vi "PH_Timing.Update Status.vi"(0 "i ref in":refnum<vi>, 5 "error in (no error)":errorcluster) -> (14 "i ref out":refnum<vi>, 19 "error out":errorcluster)   [LabVIEW 2014, in "PH_Timing.lvlib"]
doc: "By this VI the status of the timing instance is calculated, written to own attributes and published as DIM service. Additionally other services are updated.\n\n0 (no info): one or more child instances missed\n1 (off): instance started, all child instances available\n2 (on): ready to shot\n\nAdditionally the GUI elements are set."
uses:
  PH_Timing.lvlib
  PH_Basics/PH_StatusHandler/PH_StatusHandler.Status.ctl
  PH_Basics/PH_StatusHandler/PH_StatusHandler.lvlib
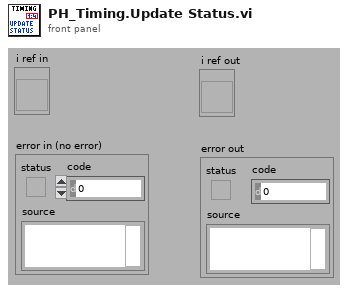
[diagram p1: front panel]
types:
  T1 = enum16{"Normal", "Single", "Burst", "Duty Cycle"}
  T2 = typedef "PH_StatusHandler.lvlib/PH_StatusHandler.Status.ctl" = i16
  T3 = typedef "PH_Timing.lvlib/PH_Timing.i attribute.ctl" = cluster{"Sequencer":cluster{"linked?":bool, "Proc State":string, "Ref State":refnum<vi>}, "Gate Generator":cluster{"GD":cluster{"Device Status":T2, "linked?":bool}, "Settings":T4, "GUI Ref":refnum<vi>}, "Interlock Bypass":cluster{"Instancename":string, "Switch linked?":bool, "Device Status":T2, "Ref Status":refnum<vi>}, "Roughtuner":cluster{"Settings":T5, "GUI Ref":refnum<vi>, "GD":cluster{"Device Status":T2, "linked?":bool}}, "0,5Hz Gater":cluster{"Settings":T6, "GUI Ref":refnum<vi>, "GD":cluster{"Device Status":T2, "linked?":bool}}, "Slow Trigger":cluster{"Settings":T7, "GUI Ref":refnum<vi>, "Service ID Delay":i32, "Service ID Ext Trig":i32, "Wanted Settings":T7}, "Timing Mode":cluster{"Mode":T8, "GUI Ref":refnum<vi>, "Service ID T2":i32, "Service ID Mode":i32, "Wanted Mode":T8}, "ns Generator":cluster{"Settings":T9, "ns Generator Settings":refnum<vi>, "GD":cluster{"Device Status":T2, "linked?":bool}}, "Phase FEs":cluster{"Settings":T12, "GUI Ref":refnum<vi>, "Service ID Phase":i32, "Wanted Settings":T12}, "GD GUI Refs":refnum<vi>[], "Heads":T13[], "GUI Ref Delete":refnum<vi>}
  T4 = typedef "PH_Timing.lvlib/PH_Timing.GateGen.ctl" = cluster{"Instance":string, "Channel Gate":i32, "Channel T2":i32, "Width Gate":dbl, "Width T2":dbl, "Delay Gate":dbl, "Delay T2":dbl, "Gate activ":bool, "T2 activ":bool, "System Mode":enum16{"Normal", "Single", "Burst", "Duty Cycle"}}
  T5 = typedef "PH_Timing.lvlib/PH_Timing.Roughtuner.ctl" = cluster{"Instance":string, "Phase PHELIX / UNILAC":cluster{"Channel":u16, "relative to":u16, "Delay [ms]":dbl}, "Pulse Length":cluster{"Channel":u16, "relative to":u16, "Delay [ms]":dbl}, "Trigger":cluster{"externally?":bool, "Rate [Hz]":dbl}}
  T6 = typedef "PH_Timing.lvlib/PH_Timing.0.5HzGater.ctl" = cluster{"Instance":string, "Channel ns FE Delay":i32, "Channel 0.5Hz":i32, "Width ns FE Delay":dbl, "Width 0.5Hz":dbl, "Delay ns FE Delay":dbl, "Delay 0.5Hz":dbl, "ns FE Delay active":bool, "0.5Hz activ":bool, "ns FE Delay inverted":bool, "0.5Hz inverted":bool}
  T7 = typedef "PH_Timing.lvlib/PH_Timing.Slow Trigger Settings.ctl" = cluster{"Delay":dbl, "externally triggered?":bool}
  T8 = typedef "PH_Timing.lvlib/PH_Timing.Timing Mode.ctl" = cluster{"T2":i16, "Modeselector":enum32{"10 Hz", "0.5 Hz", "Shot"}}
  T9 = typedef "PH_Timing.lvlib/PH_Timing.ns Generator.ctl" = cluster{"Instance":string, "Phase fs / ns FE":cluster{"Channel":T10, "Settings":T11}}
  T10 = typedef "Stanford Research DG645 - Driver.lvlib/Channel.ctl" = i32
  T11 = typedef "PH_SRDG645.lvlib/PH_SRDG645.Channel Settings.ctl" = cluster{"Delay [s]":dbl, "relative to":i32}
  T12 = typedef "PH_Timing.lvlib/PH_Timing.Phase FEs.ctl" = cluster{"Phase":dbl}
  T13 = typedef "PH_Timing.lvlib/PH_Timing.PU Data.ctl" = cluster{"linked?":bool, "Data":T14, "GD":cluster{"Device Status":T2, "linked?":bool}, "GUI Ref":refnum<vi>, "PU":T15}
  T14 = typedef "PH_Timing.lvlib/PH_Timing.PU Info.ctl" = cluster{"Act CH?":bool, "GD":string, "CH":i32, "Delay":dbl, "active":bool, "in Use?":bool}
  T15 = typedef "PH_PP_Common.lvlib/PH_PP_Common.PUs.ctl" = enum16{"no Info", "PA-19mm-1", "PA-19mm-2", "PA-45mm-PILC", "PA-45mm-MAIN", "MA-PU-1", "MA-PU-2", "MA-PU-3", "MA-PU-4", "MA-PU-5", "MA-PU-6", "MA-FR", "MA-PILC", "PA-45mm-DP"}
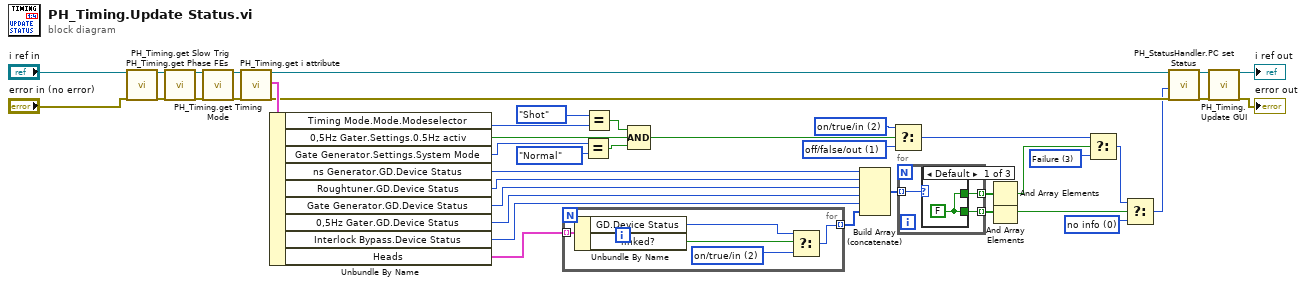
[diagram p0: block diagram]
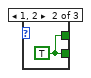
[diagram p2: hidden frame]
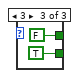
[diagram p3: hidden frame]
diagram:
  w21 = T2 1 items=["no info", "off/false/out", "on/true/in", "Failure", "Alarm", "Status 1", "Status 2", "Status 3"] ("Status.Device Status")
  w26 = T2 3 items=["no info", "off/false/out", "on/true/in", "Failure", "Alarm", "Status 1", "Status 2", "Status 3"] ("Status.Device Status")
  w23 = T2 2 items=["no info", "off/false/out", "on/true/in", "Failure", "Alarm", "Status 1", "Status 2", "Status 3"] ("Status.Device Status")
  w29 = T2 0 items=["no info", "off/false/out", "on/true/in", "Failure", "Alarm", "Status 1", "Status 2", "Status 3"] ("Status.Device Status")
  n1 = call "PH_Timing.get Phase FEs.vi"("i ref in"="i ref in", "error in"="error in (no error)") -> ("i ref out"=w32:refnum<vi>, "error out"=w31:errorcluster)  [unwired: 16 in]
  n2 = call "PH_Timing.get Slow Trig.vi"("i ref in"=w32, "error in"=w31) -> ("i ref out"=w36:refnum<vi>, "error out"=w34:errorcluster)  [unwired: 16 in]
  n3 = call "PH_Timing.get Timing Mode.vi"("i ref in"=w36, "error in"=w34) -> ("i ref out"=w35:refnum<vi>, "error out"=w33:errorcluster)  [unwired: 16 in]
  n4 = call "PH_Timing.get i attribute.vi"("i ref in"=w35, "error in (no error)"=w33) -> ("i ref out"=w40:refnum<vi>, "i attribute"=w42:T3, "error out"=w41:errorcluster)  [unwired: 15 in]
  n5 = Unbundle By Name(w42) -> ("Timing Mode.Mode.Modeselector"=w9:enum32{"10 Hz", "0.5 Hz", "Shot"}, "0,5Hz Gater.Settings.0.5Hz activ"=w20:bool, "Gate Generator.Settings.System Mode"=w19:T1, "ns Generator.GD.Device Status"=w16:T2, "Roughtuner.GD.Device Status"=w13:T2, "Gate Generator.GD.Device Status"=w12:T2, "0,5Hz Gater.GD.Device Status"=w11:T2, "Interlock Bypass.Device Status"=w7:T2, "Heads"=w4:T13[])
  n6 = for {
    tunnel: w4 -> [w47] mode=indexing
    tunnel: [w44] -> w5 mode=indexing
    w43 = T2 2 items=["no info", "off/false/out", "on/true/in", "Failure", "Alarm", "Status 1", "Status 2", "Status 3"] ("f")
    n7 = Unbundle By Name(w47) -> ("GD.Device Status"=w45:T2, "linked?"=w46:bool)
    n8 = Select(t=w45, s=w46, f=w43) -> (s? t:f=w44:T2)
  }
  n9 = Equal?(x=w19, y=T1."Normal" ("Gate Generator.Settings.System Mode")) -> (x = y?=w17:bool)
  n10 = Equal?(x=enum32{"10 Hz", "0.5 Hz", "Shot"}."Shot" ("Timing Mode.Mode.Modeselector"), y=w9) -> (x = y?=w25:bool)
  n11 = Compound Arithmetic op=AND(w25, w20, w17) -> (w24:bool)
  n12 = Build Array (concatenate)(w16, w13, w12, w11, w7, w5) -> (w14:T2[])
  n13 = Select(t=w23, s=w24, f=w21) -> (s? t:f=w22:T2)
  n14 = for {
    tunnel: [w49] -> w15 mode=indexing
    tunnel: w14 -> [w50] mode=indexing
    tunnel: [w48] -> w8 mode=indexing
    n15 = case shown="Default" w50 {
      tunnel: [w51 w52 TRUE] -> w49
      tunnel: [w51 w52 FALSE] -> w48
      frame Default {
        w51 = FALSE
      }
      frame 1, 2 {
        w52 = TRUE
      }
      frame 3 {
      }
    }
  }
  n16 = And Array Elements(Boolean array=w8) -> (logical AND=w6:bool)
  n17 = And Array Elements(Boolean array=w15) -> (logical AND=w3:bool)
  n18 = Select(t=w22, s=w6, f=w26) -> (s? t:f=w27:T2)
  n19 = Select(t=w27, s=w3, f=w29) -> (s? t:f=w28:T2)
  n20 = call "PH_StatusHandler.PC set Status.vi"("i ref in"=w40, "Status"=w28, "error in (no error)"=w41) -> ("i ref out"=w2:refnum<vi>, "error out"=w1:errorcluster)  [unwired: 15 in]
  n21 = call "PH_Timing.Update GUI.vi"("i ref in"=w2, "error in (no error)"=w1) -> ("i ref out"=→"i ref out":refnum<vi>, "error out"=→"error out":errorcluster)  [unwired: 16 in]
